vi "Creators Status Created Events.vi"(11 "Base Event in":refnum<class "Base Event.lvclass">) -> (0 "Created Event Count":i32, 1 "Created Event Aliases":string[](array[string]), 2 "Created Event Exist?":bool, 3 "Base Event out":refnum<class "Base Event.lvclass">)   [LabVIEW 2021, in "jettl.lvlib" / "Base Event.lvlib" / "Base Event.lvclass"]
uses:
  Base Event.lvclass
  C:/git/jettl/jettl/jettl/jettl/jettl.lvclass
  Base Event.lvclass/Base Event.ctl
  Addresses/Addresses.lvlib
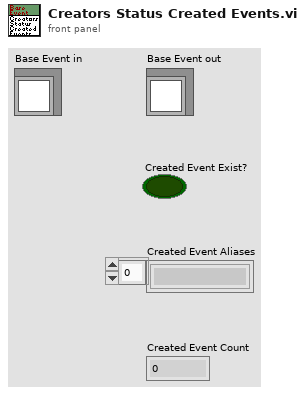
[diagram p1: front panel]
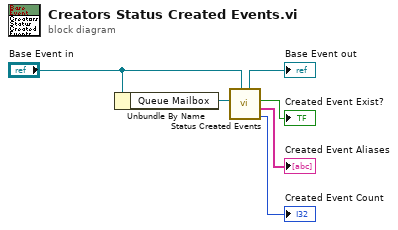
[diagram p0: block diagram]
diagram:
  n1 = Unbundle By Name("Base Event in") -> ("Queue Mailbox"=w5:refnum<data-value>)
  n2 = call "Status Created Events.vi"("jettl in"="Base Event in", "Queue Mailbox"=w5) -> ("Created Event Count"=→"Created Event Count":i32, "Created Event Aliases"=→"Created Event Aliases":string[], "Created Event Exist?"=→"Created Event Exist?":bool, "jettl out"=→"Base Event out":refnum<class "Base Event.lvclass">)  [unwired: 6 in]
